vi "Process module.vi"(6 "start pixel":i32, 7 "Action":string, 8 "error in":errorcluster, 9 "#pixels to save":i32=200, 10 "#A-lines to save":i32=2048, 11 "Save":bool) -> (0 "Error Out":errorcluster, 2 "Exit?":bool, 3 "# elements in save queue":i32)   [LabVIEW 2018]
uses:
  Controls/Queue Manager Actions.ctl
  Controls/QueueNames.ctl
  Controls/MessagePacket.ctl
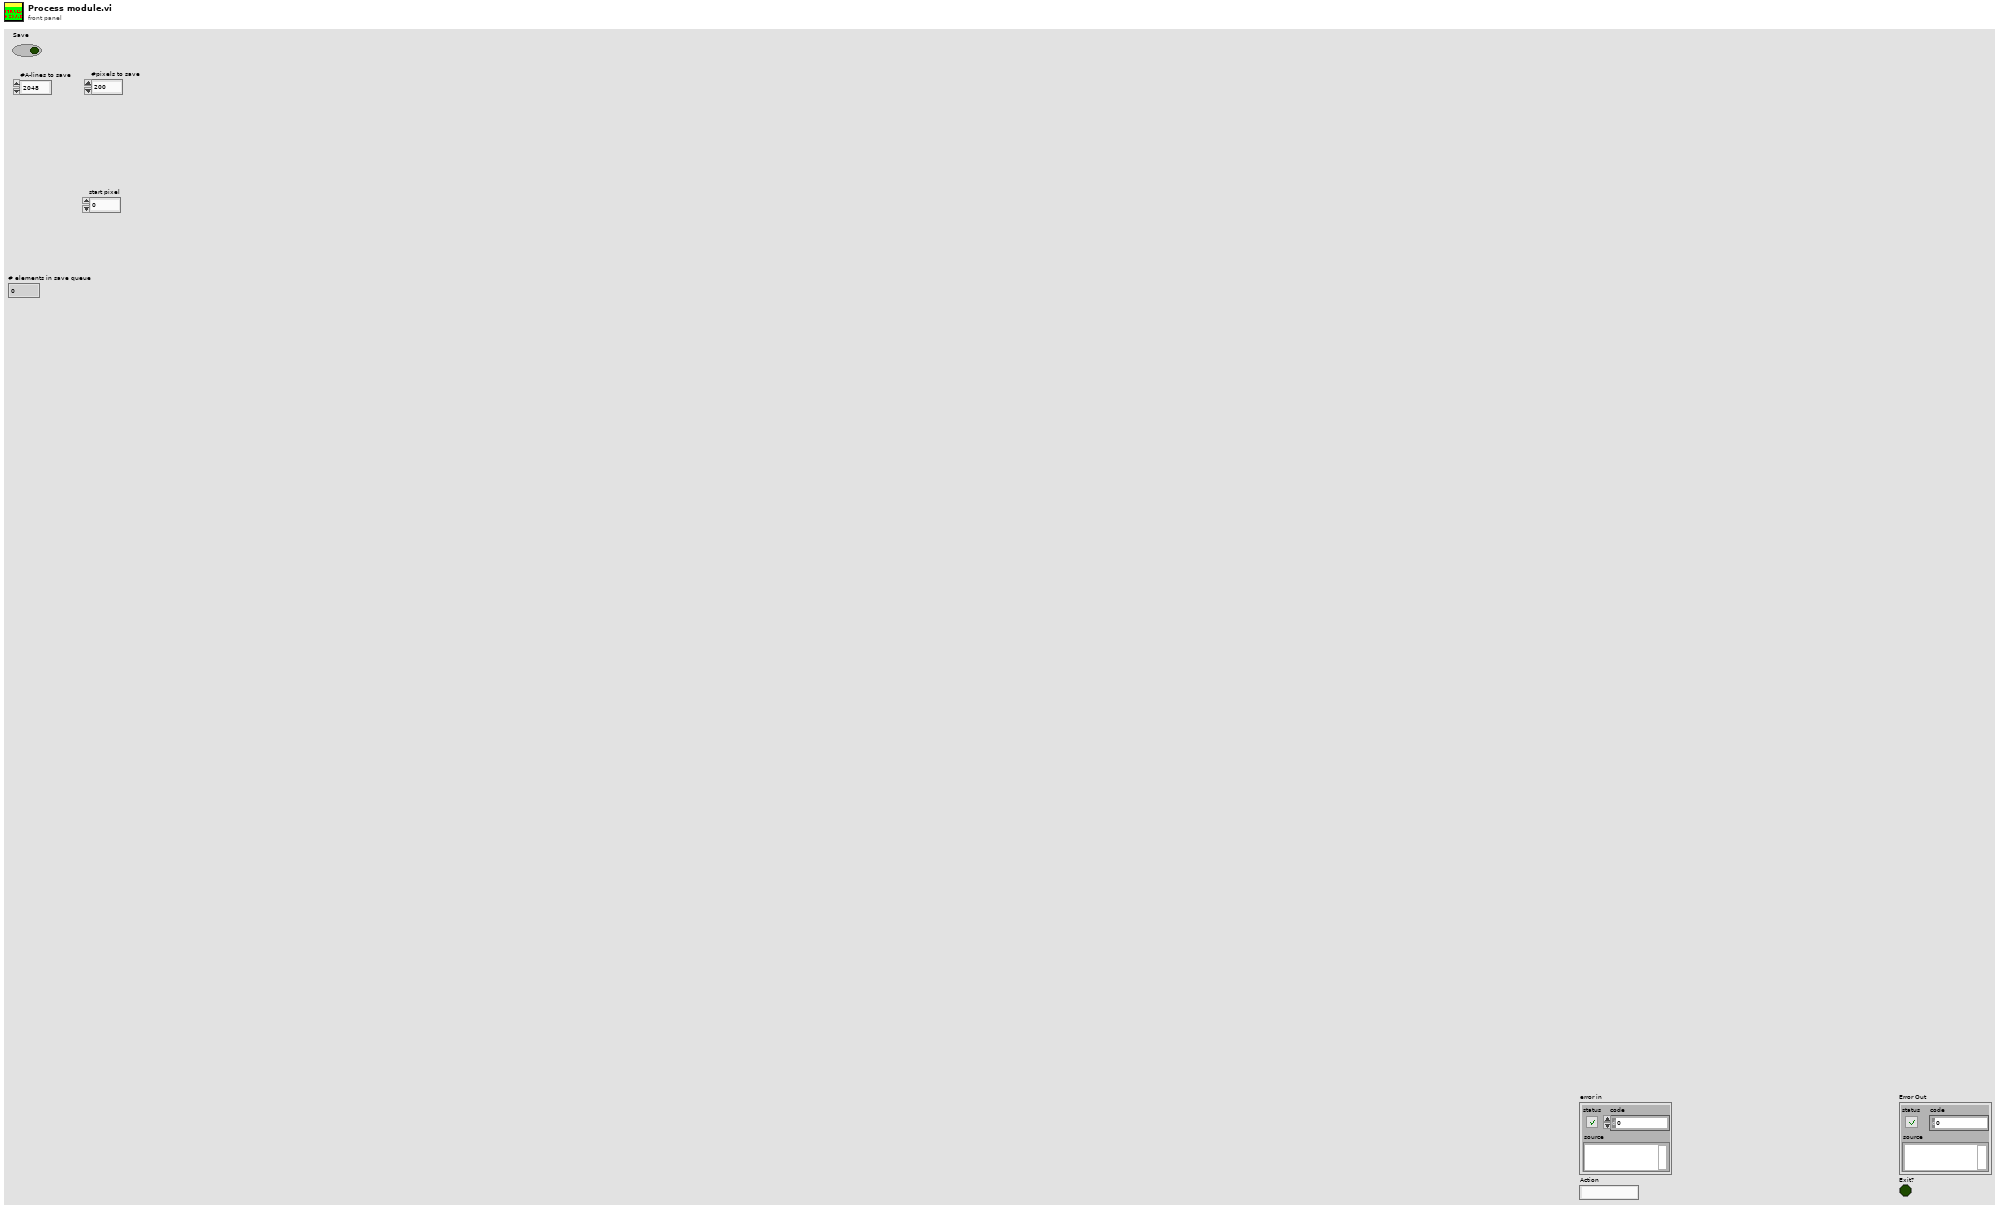
[diagram p1: front panel]
types:
  T1 = typedef "Queue Manager Actions.ctl" = enum16{"Init", "Enqueue", "Enqueue All", "Preview Queue", "Dequeue", "Get Status", "Flush Queue", "Flush All Queues", "Release All Queues", "Release Queue", "Enqueue at Opposite End"}
  T2 = typedef "MessagePacket.ctl" = cluster{"Message":string, "Parameter":variant}
  T3 = typedef "QueueNames.ctl" = enum16{"Main GUI", "Main Scan Processor", "Main Processing", "Main Saving", "Main Display", "Main Table Stage GUI", "Main Table Stage Proc.", "Scan Engine", "Vibratome GUI", "Vibratome Processor", "Slice Engine"}
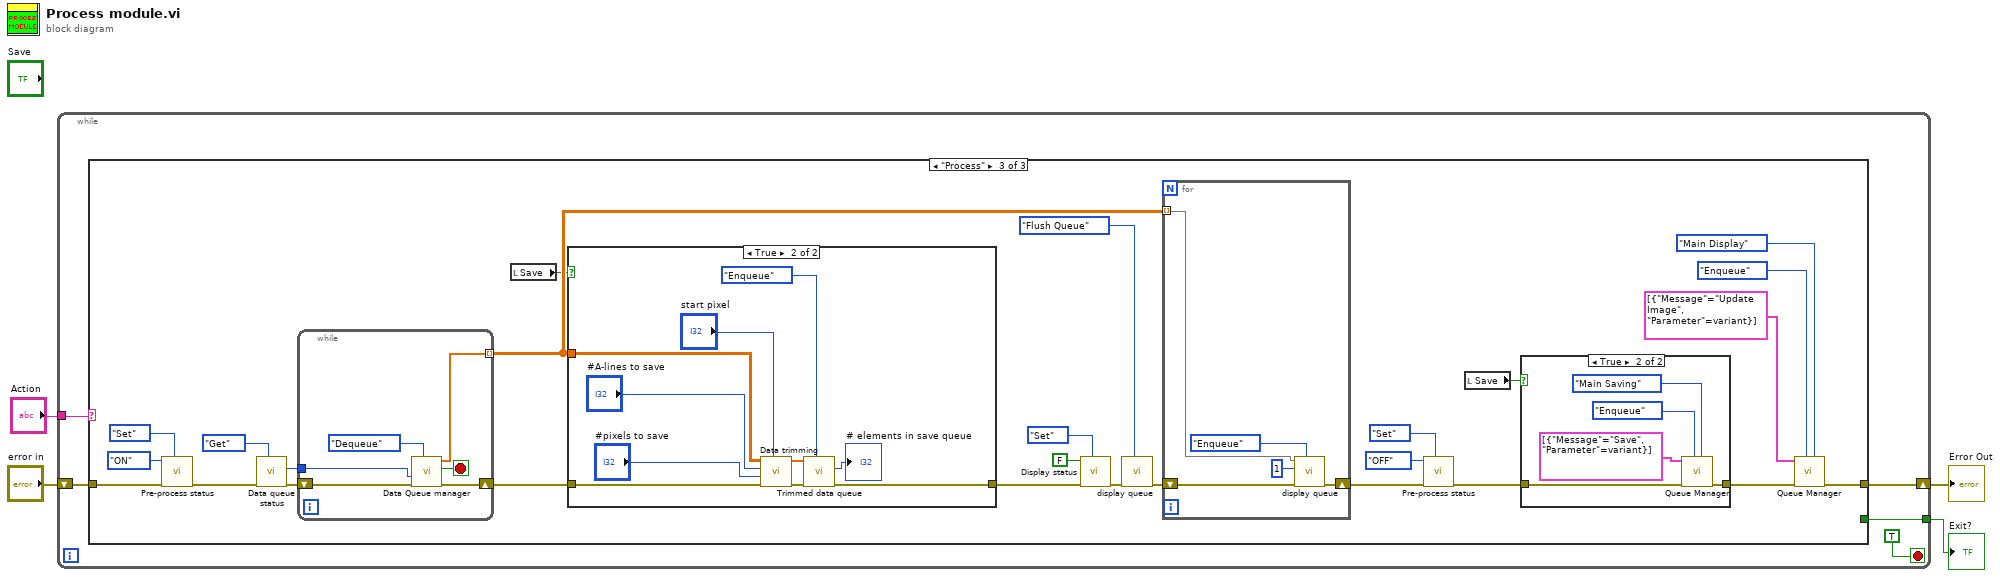
[diagram p0: block diagram]
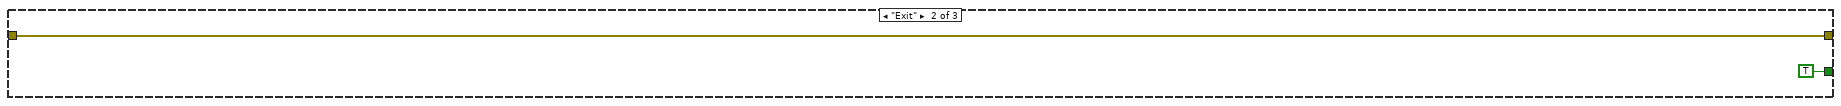
[diagram p3: hidden frame]
diagram:
  n1 = while {
    tunnel: "Action" -> [w7]
    shift-right: [w8] -> w3
    shift-left: "error in" -> [w9]
    tunnel: [w5] -> w1
    stop <- TRUE stop-if-true
    n2 = case shown="\"Process\"" w7 {
      tunnel: w9 -> [w10 w11 w17]
      tunnel: [w10 w11 w16] -> w8
      tunnel: [_ TRUE _] -> w5
      frame "Init", Default {
      }
      frame "Exit" {
      }
      frame "Process" {
        n3 = call "Pre-process status.vi"("action"=enum16{"Init", "Get", "Set"}."Set", "error in"=w17, "pre-processing status in"=enum16{"ON", "OFF"}."ON") -> ("error out"=w23:errorcluster)  [unwired: 7 in, 1 out]
        n4 = call "Data queue status.vi"("action"=enum16{"Init", "Get", "Set"}."Get", "error in"=w23) -> ("error out"=w22:errorcluster, "dequeue channel"=w20:enum16{"1", "2"})  [unwired: 7 in, 1 out]
        n5 = while {
          tunnel: [w64] -> w19 mode=indexing
          shift-right: [w62] -> w38
          shift-left: w22 -> [w65]
          tunnel: w20 -> [w61]
          stop <- w66 stop-if-true
          n6 = call "Data Queue manager.vi"("Action"=Queue_Manager_Actions."Dequeue", "error in"=w65, "dequeue channel"=w61) -> ("error out"=w62:errorcluster, "Empty?"=w66:bool, "data out"=w64:sgl[])  [unwired: 5 in, 1 out]
        }
        n7 = local read "Save"() -> (w18:bool)
        n8 = case shown="True" w18 {
          tunnel: w38 -> [w44 w54]
          tunnel: [w44 w53] -> w15
          tunnel: w19 -> [_ w52]
          frame False {
          }
          frame True {
            n9 = call "Data trimming.vi"("start pixel"="start pixel", "error in"=w54, "#pixels to save"="#pixels to save", "#A-lines"="#A-lines to save", "2D Array in"=w52) -> ("error out"=w47:errorcluster, "array for saving"=w51:sgl[])  [unwired: 4 in, 1 out]
            n10 = call "Trimmed data queue.vi"("Action"=Queue_Manager_Actions."Enqueue", "error in (no error)"=w47, "data in"=w51) -> ("error out"=w53:errorcluster, "# elements in queue"=→"# elements in save queue":i32)  [unwired: 5 in, 2 out]
          }
        }
        n11 = call "Display status.vi"("action"=enum16{"Init", "Get", "Set"}."Set", "error in"=w15, "display status in"=FALSE) -> ("error out"=w24:errorcluster)  [unwired: 7 in, 1 out]
        n12 = call "display queue.vi"("Action"=Queue_Manager_Actions."Flush Queue", "error in (no error)"=w24) -> ("error out"=w13:errorcluster)  [unwired: 5 in, 4 out]
        n13 = for {
          tunnel: w19 -> [w39] mode=indexing
          shift-right: [w42] -> w37
          shift-left: w13 -> [w43]
          n14 = call "display queue.vi"("Action"=Queue_Manager_Actions."Enqueue", "error in (no error)"=w43, "time out"=1, "input data"=w39) -> ("error out"=w42:errorcluster)  [unwired: 3 in, 4 out]
        }
        n15 = call "Pre-process status.vi"("action"=enum16{"Init", "Get", "Set"}."Set", "error in"=w37, "pre-processing status in"=enum16{"ON", "OFF"}."OFF") -> ("error out"=w31:errorcluster)  [unwired: 7 in, 1 out]
        n16 = local read "Save"() -> (w29:bool)
        n17 = case shown="True" w29 {
          tunnel: w31 -> [w55 w57]
          tunnel: [w55 w56] -> w30
          frame False {
          }
          frame True {
            n18 = call "Queue Manager.vi"("Queue Name"=QueueNames."Main Saving", "Action"=Queue_Manager_Actions."Enqueue", "Error In"=w57, "Message Packet Array"=T2[] [{"Message"="Save", "Parameter"=variant}]) -> ("Error Out"=w56:errorcluster)  [unwired: 3 in, 4 out]
          }
        }
        n19 = call "Queue Manager.vi"("Queue Name"=QueueNames."Main Display", "Action"=Queue_Manager_Actions."Enqueue", "Error In"=w30, "Message Packet Array"=T2[] [{"Message"="Update Image", "Parameter"=variant}]) -> ("Error Out"=w16:errorcluster)  [unwired: 3 in, 4 out]
      }
    }
  }
  "Error Out" <- w3
  "Exit?" <- w1
